vi "Open File Count.vi"(8 "error in (no error)":errorcluster, 11 "Excel Interface in":refnum<class "Excel Interface.lvclass">) -> (0 "error out":errorcluster, 2 "Count":i32, 3 "Excel Interface out":refnum<class "Excel Interface.lvclass">)   [LabVIEW 2013, in "Excel Interface.lvclass"]
uses:
  Excel Interface.lvclass
  Excel Interface.lvclass/Excel Interface.ctl
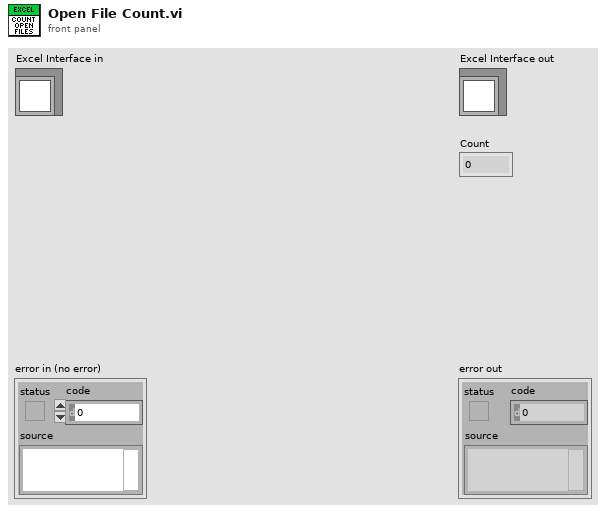
[diagram p1: front panel]
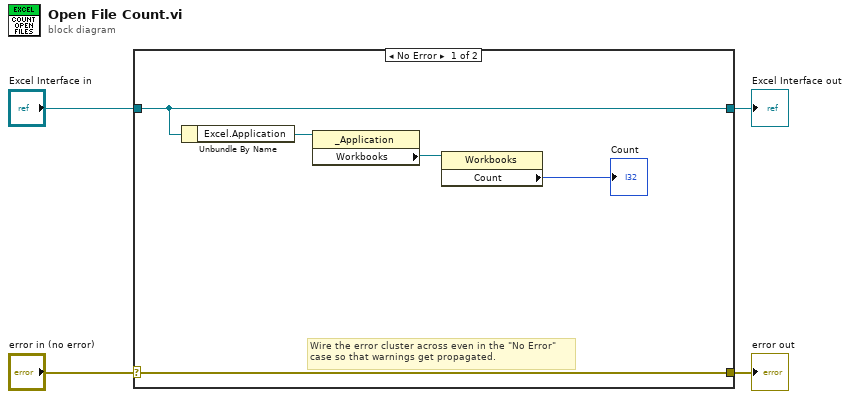
[diagram p0: block diagram]
diagram:
  n1 = case shown="No Error" "error in (no error)" {
    selector: "error in (no error)" -> [w9 w11]
    tunnel: [w9 w11] -> w3
    tunnel: [w8 w10] -> w1
    tunnel: "Excel Interface in" -> [w8 w10]
    frame No Error {
      # "Wire the error cluster across even in the \"No Error\"\ncase so that warnings get propagated."
      n2 = Unbundle By Name(w8) -> ("Excel.Application"=w7:refnum<k7>)
      n3 = property class="_Application"(reference=w7) -> ("Workbooks"=w6:refnum<k7>)  [unwired: 1 in, 2 out]
      n4 = property class="Workbooks"(reference=w6) -> ("Count"=→"Count":i32)  [unwired: 1 in, 2 out]
    }
    frame Error {
    }
  }
  "error out" <- w3
  "Excel Interface out" <- w1
